vi "Pull_Data_via_Public_Client.vi"(2 "application reference":refnum<vi>, 3 "error in (no error)":errorcluster, 4 "Archive Files?":bool, 5 "Running on Server?":bool, 6 "Path of File relative to EnFlo Data Root":path[](array[path])) -> (0 "error out":errorcluster)   [LabVIEW 2012]
uses:
  Anemometry/Anemometry Sub Vis/Globals/Constants_global.vi
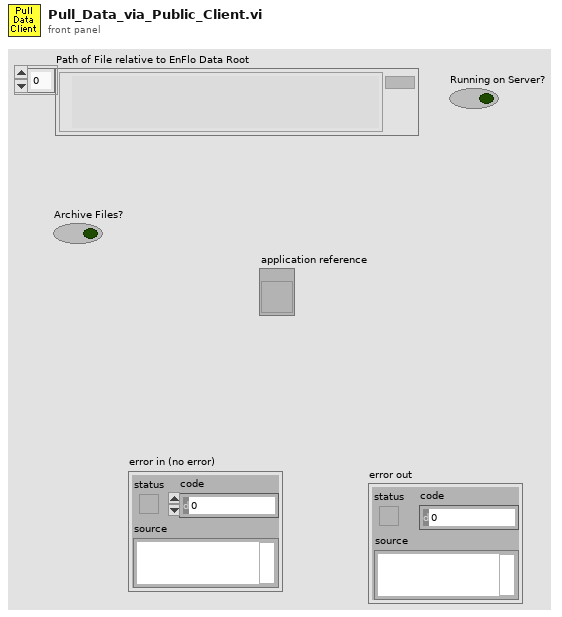
[diagram p1: front panel]
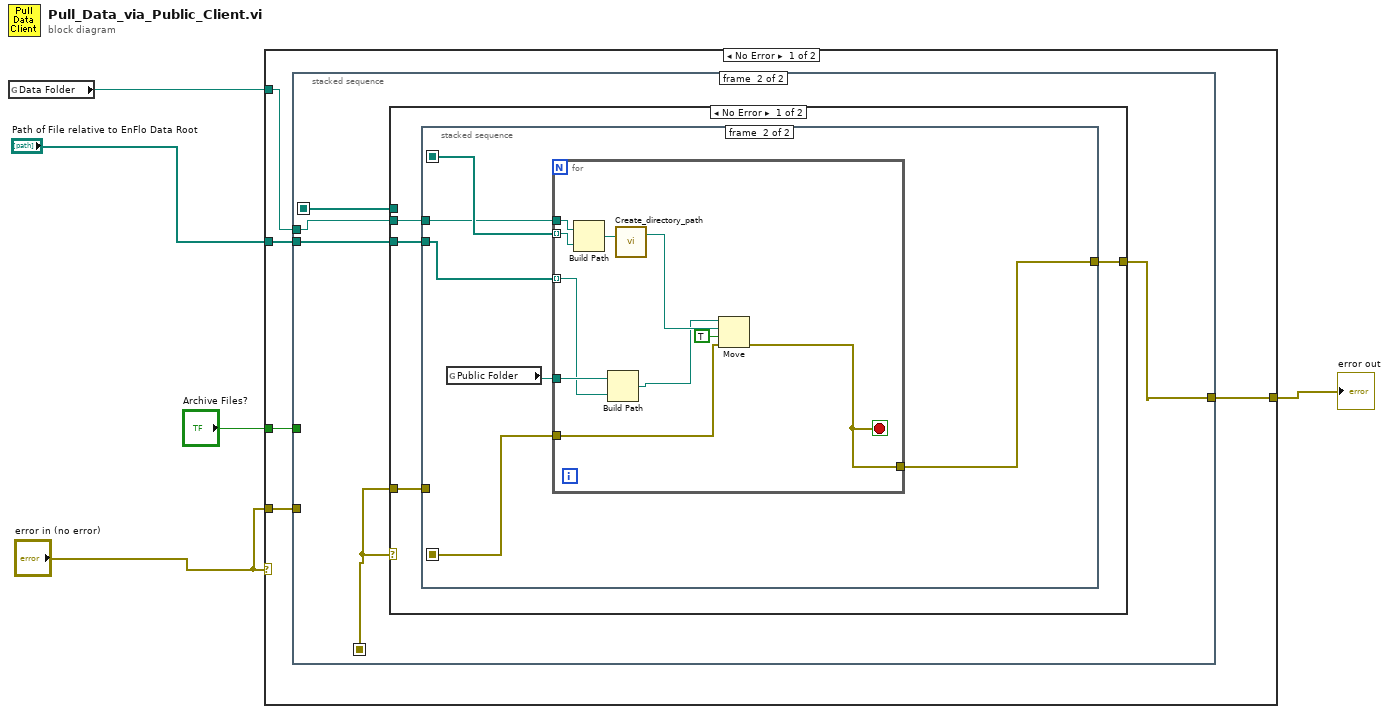
[diagram p0: block diagram]
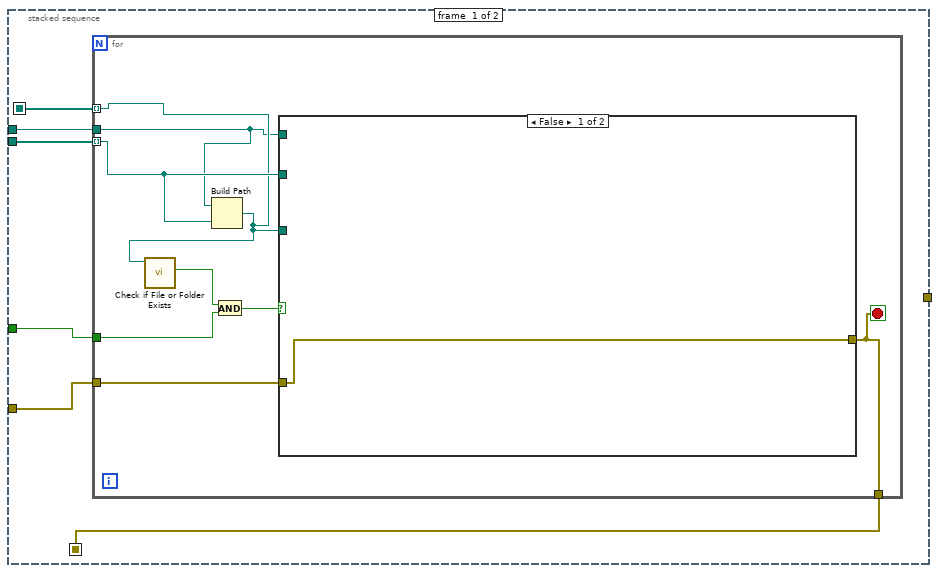
[diagram p2: hidden frame]
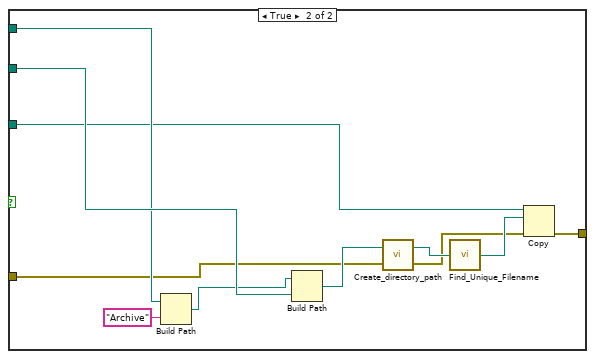
[diagram p3: hidden frame]
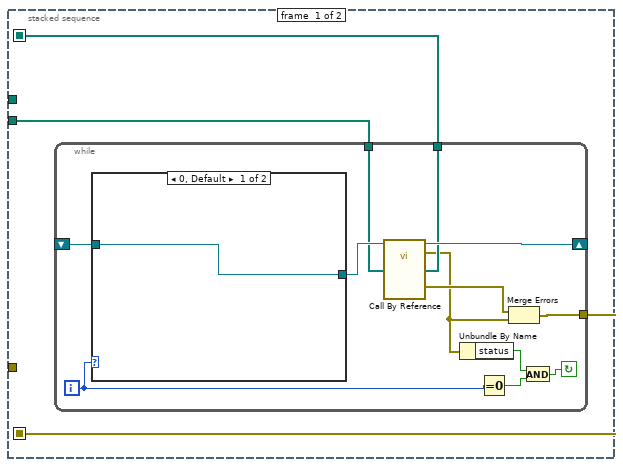
[diagram p4: hidden frame]
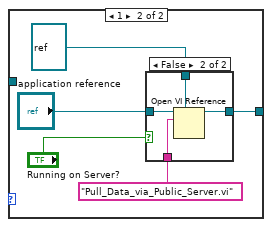
[diagram p5: hidden frame]
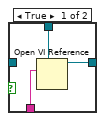
[diagram p6: hidden frame]
diagram:
  n1 = global read "Constants_global.vi" "Data Folder"() -> (w1:path)
  n2 = case shown="No Error" "error in (no error)" {
    tunnel: [w10 w91] -> w3
    tunnel: "error in (no error)" -> [w9 w91]
    tunnel: "Path of File relative to EnFlo Data Root" -> [w8 _]
    tunnel: "Archive Files?" -> [w7 _]
    tunnel: w1 -> [w6 _]
    frame No Error {
      n3 = stacked-sequence {
        seq-local: [w15 _] -> [_ w38]
        seq-local: [w13 _] -> [_ w40]
        tunnel: [_ w41] -> w10
        tunnel: w9 -> [w16 _]
        tunnel: w8 -> [w14 w39]
        tunnel: w7 -> [w12 _]
        tunnel: w6 -> [w11 w37]
        frame #0 {
          n4 = for {
            tunnel: w16 -> [w24]
            tunnel: [w19] -> w15
            tunnel: w14 -> [w23] mode=indexing
            tunnel: w12 -> [w22]
            tunnel: [w18] -> w13 mode=indexing
            tunnel: w11 -> [w17]
            stop <- w19 stop-if-true
            n5 = Build Path(base path=w17, name or relative path=w23) -> (appended path=w18:path)
            n6 = call <vilib>:"Check if File or Folder Exists.vi"("path"=w18) -> ("file or folder exists?"=w21:bool)  [unwired: 8 in, 2 out]
            n7 = And(x=w21, y=w22) -> (x .and. y?=w20:bool)
            n8 = case shown="False" w20 {
              tunnel: w17 -> [_ w30]
              tunnel: w23 -> [_ w32]
              tunnel: [w25 w28] -> w19
              tunnel: w24 -> [w25 w27]
              tunnel: w18 -> [_ w26]
              frame False {
              }
              frame True {
                n9 = Build Path(base path=w30, name or relative path="Archive") -> (appended path=w29:path)
                n10 = Build Path(base path=w29, name or relative path=w32) -> (appended path=w35:path)
                n11 = call "Create_directory_path.vi"("error in (no error)"=w27, "Path name"=w35) -> ("error out"=w33:errorcluster, "Path name Out"=w34:path)
                n12 = call "Find_Unique_Filename.vi"("Path In"=w34) -> ("Unique Path Out"=w36:path)  [unwired: 2 in]
                n13 = Copy(8:w33, 10:w36, 11:w26) -> (0:w28:errorcluster)  [unwired: 2 in, 2 out]
              }
            }
          }
        }
        frame #1 {
          n14 = case shown="No Error" w38 {
            tunnel: [w43 w90] -> w41
            tunnel: w38 -> [w44 w90]
            tunnel: w40 -> [_ _]
            tunnel: w39 -> [w45 _]
            tunnel: w37 -> [w42 _]
            frame No Error {
              n15 = stacked-sequence {
                seq-local: [w47 _] -> [_ w79]
                seq-local: [w46 _] -> [_ w75]
                tunnel: w45 -> [w48 w77]
                tunnel: w44 -> [_ _]
                tunnel: [_ w76] -> w43
                tunnel: w42 -> [_ w74]
                frame #0 {
                  n16 = while {
                    shift-right: [w58] -> _
                    shift-left: _ -> [w60]
                    tunnel: w48 -> [w53]
                    tunnel: [w52] -> w47
                    tunnel: [w49] -> w46
                    i -> [w57]
                    stop <- w54 continue-if-true
                    n17 = case shown="0, Default" w57 {
                      tunnel: w60 -> [w61 _]
                      tunnel: [w61 w66] -> w59
                      frame 0, Default {
                      }
                      frame 1 {
                        n18 = case shown="False" "Running on Server?" {
                          tunnel: [w69 w73] -> w66
                          tunnel: "application reference" -> [_ w72]
                          tunnel: refnum<vi> refnum ("Push Data Server") -> [w68 w71]
                          tunnel: "Pull_Data_via_Public_Server.vi" -> [w67 w70]
                          frame True {
                            n19 = Open VI Reference(type specifier VI Refnum (for type only)=w68, vi path=w67) -> (vi reference=w69:refnum<vi>)  [unwired: 2 in, 3 out]
                          }
                          frame False {
                            n20 = Open VI Reference(type specifier VI Refnum (for type only)=w71, application reference (local)=w72, vi path=w70) -> (vi reference=w73:refnum<vi>)  [unwired: 1 in, 3 out]
                          }
                        }
                      }
                    }
                    n21 = call-by-ref "?"(reference=w59, "Path of File relative to EnFlo Data Root"=w53) -> (reference out=w58:refnum<vi>, error out=w50:errorcluster, "error out"=w51:errorcluster, "Relative Paths Out"=w52:path[])  [unwired: 2 in]
                    n22 = Unbundle By Name(w50) -> ("status"=w55:bool)
                    n23 = Equal To 0?(x=w57) -> (x = 0?=w56:bool)
                    n24 = Merge Errors(w51, w50) -> (w49:errorcluster)
                    n25 = And(x=w55, y=w56) -> (x .and. y?=w54:bool)
                  }
                }
                frame #1 {
                  n26 = global read "Constants_global.vi" "Public Folder"() -> (w78:path)
                  n27 = for {
                    tunnel: w79 -> [w81] mode=indexing
                    tunnel: w78 -> [w88]
                    tunnel: w77 -> [w87] mode=indexing
                    tunnel: w75 -> [w84]
                    tunnel: [w83] -> w76
                    tunnel: w74 -> [w80]
                    stop <- w83 stop-if-true
                    n28 = Build Path(base path=w80, name or relative path=w81) -> (appended path=w82:path)
                    n29 = Build Path(base path=w88, name or relative path=w87) -> (appended path=w86:path)
                    n30 = call "Create_directory_path.vi"("Path name"=w82) -> ("Path name Out"=w89:path)  [unwired: 1 in, 1 out]
                    n31 = Move(source path=w86, error in=w84, 9:TRUE ("overwrite (F)"), 10:w89) -> (error out=w83:errorcluster)  [unwired: 1 in, 2 out]
                  }
                }
              }
            }
            frame Error {
            }
          }
        }
      }
    }
    frame Error {
    }
  }
  "error out" <- w3
